vi "Directory Contents Copy.vi"(8 "error in":errorcluster, 9 "overwrite (F)":bool, 10 "Destination Folder":path, 11 "Source Folder":path) -> (0 "error out":errorcluster)   [LabVIEW 2020]
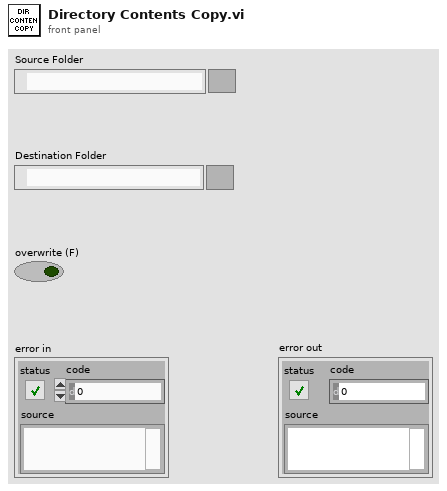
[diagram p1: front panel]
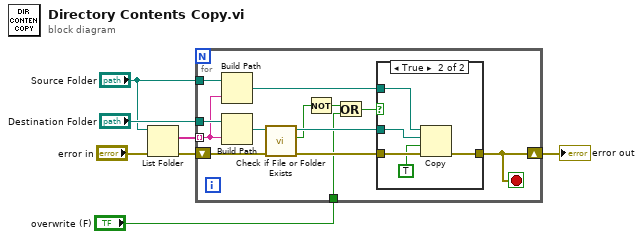
[diagram p0: block diagram]
diagram:
  n1 = List Folder(path="Source Folder", error in="error in") -> (filenames=w5:string[], error out=w3:errorcluster)  [unwired: 2 in, 2 out]
  n2 = for {
    tunnel: w5 -> [w17] mode=indexing
    tunnel: "Source Folder" -> [w20]
    shift-right: [w16] -> w4
    shift-left: w3 -> [w15]
    tunnel: "Destination Folder" -> [w18]
    tunnel: "overwrite (F)" -> [w9]
    stop <- w16 stop-if-true
    n3 = Build Path(base path=w20, name or relative path=w17) -> (appended path=w19:path)
    n4 = Build Path(base path=w18, name or relative path=w17) -> (appended path=w13:path)
    n5 = call <vilib>:"Check if File or Folder Exists.vi"("error in (no error)"=w15, "path"=w13) -> ("error out"=w14:errorcluster, "file or folder exists?"=w11:bool, "dup path"=w12:path)  [unwired: 7 in]
    n6 = Not(x=w11) -> (.not. x?=w10:bool)
    n7 = Or(x=w10, y=w9) -> (x .or. y?=w8:bool)
    n8 = case shown="True" w8 {
      tunnel: w14 -> [w21 w26]
      tunnel: w19 -> [_ w25]
      tunnel: w12 -> [_ w24]
      tunnel: [w21 w23] -> w16
      frame False {
      }
      frame True {
        n9 = Copy(8:w26, 9:TRUE ("overwrite (F)"), 10:w24, 11:w25) -> (0:w23:errorcluster)  [unwired: 1 in, 2 out]
      }
    }
  }
  "error out" <- w4
